vi "Periodic Tasks.vi"(8 "error in":errorcluster) -> ()   [LabVIEW 2012]
doc: "This VI runs in parallel to other tasks. It can contain as many user-defined periodic loops as you need. These can carry out PID or other sorts of timed response."
uses:
  <vilib>/Rock Robotics/SystemInterfaces/Utilities/FPGA_UtilitiesLED Source.ctl
  <vilib>/Rock Robotics/SystemInterfaces/Utilities/FPGA_UtilitiesLED State.ctl
  <vilib>/Rock Robotics/WPI/Relay/WPI_RelayValue.ctl
  <vilib>/Rock Robotics/WPI/RobotDrive/WPI_RobotDriveGetSetRefNum.vi
  Robot Global Data.vi
  <vilib>/Rock Robotics/WPI/Joystick/WPI_JoystickGetSetRefNum.vi
panel:
  out "end time":dbl
  out "start time":dbl
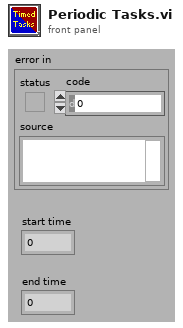
[diagram p1: front panel]
types:
  T1 = typedef "WPI_JoystickDevRef.ctl" = cluster{"Device":T2}
  T2 = typedef "WPI_JoystickDeviceEnum.ctl" = enum16{"USB 1", "USB 2", "USB 3", "USB 4", "Kinect 1", "Kinect 2"}
  T3 = typedef "WPI_RobotDriveDevRef.ctl" = cluster{"DevStatus":errorcluster, "Motors[]":T4[], "Square Inputs":bool, "Max Output":dbl, "Isochronous":bool}
  T4 = typedef "WPI_MotorControlDeviceRef.ctl" = cluster{"DeviceStatus":errorcluster, "Type":enum16{"PWM", "CAN"}, "PWM":cluster{"Digital Module":T5, "PWM Channel":T6, "DeadBand":T7}, "CAN":cluster{"Device Number":u8, "Control Mode":T8, "Semaphore":T9, "Max Vout":dbl}, "Invert":bool, "TransformRef":T10, "InvTransformRef":T10}
  T5 = typedef "FPGA_TypedefDigitalModule.ctl" = enum16{"Digital Module 1", "Digital Module 2"}
  T6 = typedef "FPGA_DIOPWMChannel.ctl" = enum8{"PWM 1", "PWM 2", "PWM 3", "PWM 4", "PWM 5", "PWM 6", "PWM 7", "PWM 8", "PWM 9", "PWM 10", "Invalid"}
  T7 = typedef "WPI_PWMDeadband.ctl" = cluster{"Name":string, "maxPositivePwm":i32, "minPositivePwm":i32, "centerPwm":i32, "maxNegativePwm":i32, "minNegativePwm":i32, "angularRange":u16}
  T8 = typedef "WPI_CANJaguar_ControlMode.ctl" = enum8{"Percent VBus", "Current", "Speed", "Position", "Voltage"}
  T9 = typedef "Semaphore RefNum" = refnum<k1>
  T10 = typedef "WPI_PWMTransform_ConPane.ctl" = refnum<vi>
  T11 = cluster{"JoystickDevRef":T1, "RobotDriveDevRef":T3}
  T12 = typedef "WPI_RelayValue.ctl" = enum16{"Off", "On", "Forward", "Reverse"}
  T13 = typedef "WPI_RelayDevRef.ctl" = cluster{"DevStatus":errorcluster, "Relay Channel":T14, "Digital Module":T5, "Relay Direction":T15}
  T14 = typedef "FPGA_DIORelayChannel.ctl" = enum8{"Relay 1", "Relay 2", "Relay 3", "Relay 4", "Relay 5", "Relay 6", "Relay 7", "Relay 8", "Invalid"}
  T15 = typedef "WPI_RelayDirection.ctl" = enum16{"Both directions", "Forward only", "Reverse only"}
  T16 = typedef "FPGA_UtilitiesLED State.ctl" = enum16{"Off", "On", "Toggle"}
  T17 = typedef "FPGA_UtilitiesLED Source.ctl" = enum16{"User LED", "FPGA LED"}
  T18 = typedef "WPI_CompressorDevRef.ctl" = cluster{"DevStatus":errorcluster, "DigitalInputDevRef":T19, "RelayDevRef":T13}
  T19 = typedef "WPI_DigitalInputDevRef.ctl" = cluster{"DevStatus":errorcluster, "DIO Channel":T20, "Digital Module":T5}
  T20 = typedef "FPGA_DIOChannel.ctl" = enum8{"DIO 1", "DIO 2", "DIO 3", "DIO 4", "DIO 5", "DIO 6", "DIO 7", "DIO 8", "DIO 9", "DIO 10", "DIO 11", "DIO 12", "DIO 13", "DIO 14", "Invalid"}
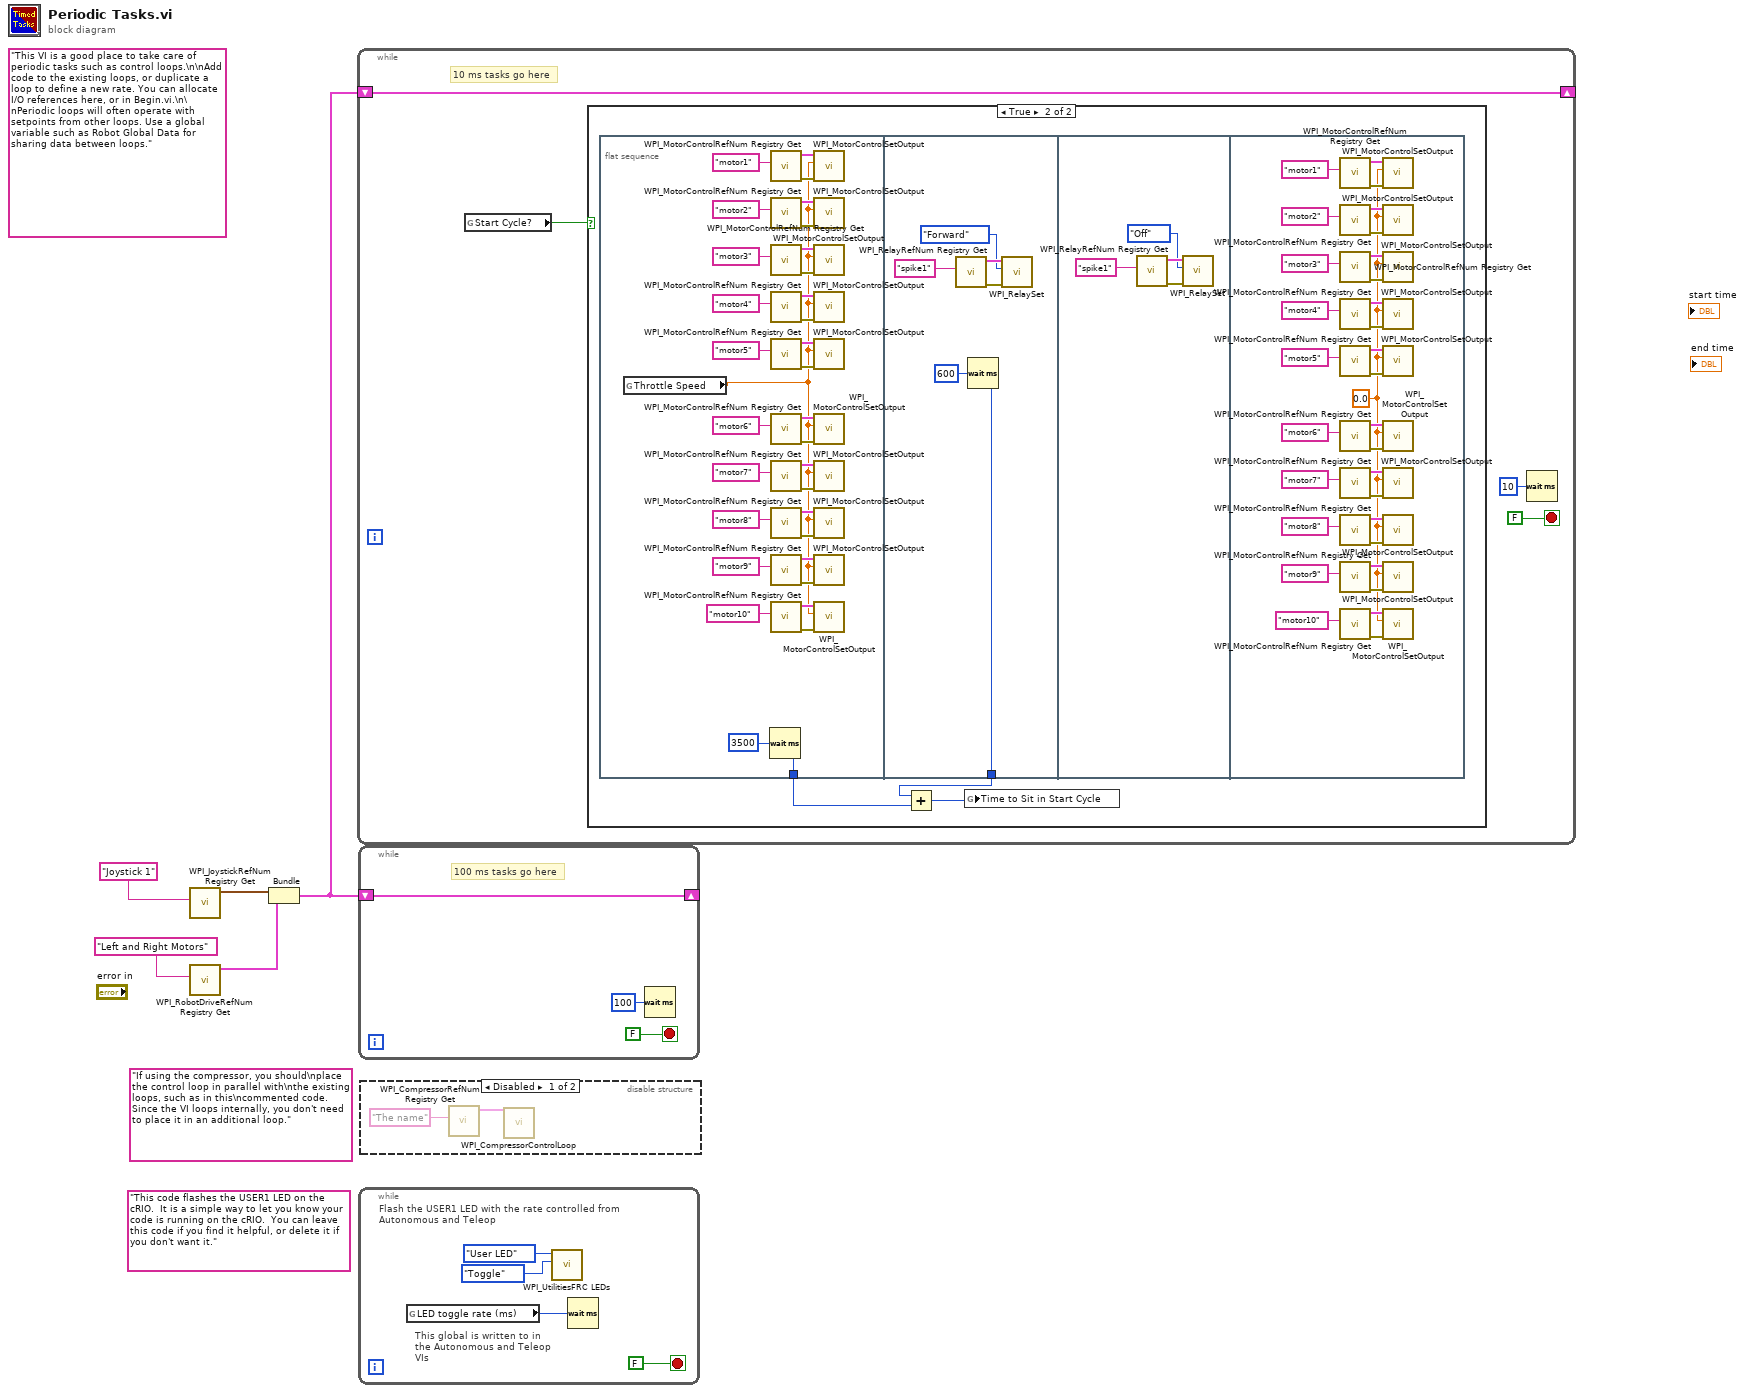
[diagram p0: block diagram]
diagram:
  (unwired) "If using the compressor, you should\nplace the control loop in parallel with\nthe existing loops, such as in this\ncommented code. Since the VI loops internally, you don't need to place it in an additional loop."
  (unwired) "This code flashes the USER1 LED on the cRIO.  It is a simple way to let you know your code is running on the cRIO.  You can leave this code if you find it helpful, or delete it if you don't want it."
  (unwired) "This VI is a good place to take care of periodic tasks such as control loops.\n\nAdd code to the existing loops, or duplicate a loop to define a new rate. You can allocate I/O references here, or in Begin.vi.\n\nPeriodic loops will often operate with setpoints from other loops. Use a global variable such as Robot Global Data for sharing data between loops."
  n1 = call <vilib>:"WPI_JoystickRefNum Registry Get.vi"("refnum name"="Joystick 1") -> ("JoystickDevRef"=w3:T1)  [unwired: 1 in, 9 out]
  n2 = call <vilib>:"WPI_RobotDriveRefNum Registry Get.vi"("refnum name"="Left and Right Motors") -> ("RobotDriveDevRef"=w2:T3)  [unwired: 1 in, 9 out]
  n3 = Bundle("JoystickDevRef"=w3, "RobotDriveDevRef"=w2) -> (w1:T11)  [unwired: 1 out]
  n4 = while {
    shift-right: [w7] -> _
    shift-left: w1 -> [w7]
    stop <- FALSE stop-if-true
    # "10 ms tasks go here"
    n5 = global read "Robot Global Data.vi" "Start Cycle?"() -> (w6:bool)
    n6 = case shown="True" w6 {
      frame False {
      }
      frame True {
        n7 = flat-sequence {
          tunnel: [w14] -> w10
          tunnel: [w46] -> w11
          frame #0 {
            n8 = global read "Robot Global Data.vi" "Throttle Speed"() -> (w13:dbl)
            n9 = Wait (ms)(milliseconds to wait=u32 3500) -> (millisecond timer value=w14:u32)
            n10 = call <vilib>:"WPI_MotorControlRefNum Registry Get.vi"("refnum name"="motor1") -> ("error out"=w40:errorcluster, "MotorControlDevRef"=w39:T4)  [unwired: 9 in]
            n11 = call <vilib>:"WPI_MotorControlRefNum Registry Get.vi"("refnum name"="motor2") -> ("error out"=w43:errorcluster, "MotorControlDevRef"=w42:T4)  [unwired: 9 in]
            n12 = call <vilib>:"WPI_MotorControlRefNum Registry Get.vi"("refnum name"="motor3") -> ("error out"=w34:errorcluster, "MotorControlDevRef"=w33:T4)  [unwired: 9 in]
            n13 = call <vilib>:"WPI_MotorControlRefNum Registry Get.vi"("refnum name"="motor4") -> ("error out"=w22:errorcluster, "MotorControlDevRef"=w21:T4)  [unwired: 9 in]
            n14 = call <vilib>:"WPI_MotorControlRefNum Registry Get.vi"("refnum name"="motor5") -> ("error out"=w25:errorcluster, "MotorControlDevRef"=w24:T4)  [unwired: 9 in]
            n15 = call <vilib>:"WPI_MotorControlRefNum Registry Get.vi"("refnum name"="motor6") -> ("error out"=w28:errorcluster, "MotorControlDevRef"=w27:T4)  [unwired: 9 in]
            n16 = call <vilib>:"WPI_MotorControlRefNum Registry Get.vi"("refnum name"="motor7") -> ("error out"=w16:errorcluster, "MotorControlDevRef"=w15:T4)  [unwired: 9 in]
            n17 = call <vilib>:"WPI_MotorControlRefNum Registry Get.vi"("refnum name"="motor8") -> ("error out"=w19:errorcluster, "MotorControlDevRef"=w18:T4)  [unwired: 9 in]
            n18 = call <vilib>:"WPI_MotorControlRefNum Registry Get.vi"("refnum name"="motor9") -> ("error out"=w37:errorcluster, "MotorControlDevRef"=w36:T4)  [unwired: 9 in]
            n19 = call <vilib>:"WPI_MotorControlRefNum Registry Get.vi"("refnum name"="motor10") -> ("error out"=w31:errorcluster, "MotorControlDevRef"=w30:T4)  [unwired: 9 in]
            n20 = call <vilib>:"WPI_MotorControlSetOutput.vi"("error in (no error)"=w40, "Output"=w13, "MotorControlDevRef"=w39) -> ()  [unwired: 6 in, 3 out]
            n21 = call <vilib>:"WPI_MotorControlSetOutput.vi"("error in (no error)"=w43, "Output"=w13, "MotorControlDevRef"=w42) -> ()  [unwired: 6 in, 3 out]
            n22 = call <vilib>:"WPI_MotorControlSetOutput.vi"("error in (no error)"=w34, "Output"=w13, "MotorControlDevRef"=w33) -> ()  [unwired: 6 in, 3 out]
            n23 = call <vilib>:"WPI_MotorControlSetOutput.vi"("error in (no error)"=w22, "Output"=w13, "MotorControlDevRef"=w21) -> ()  [unwired: 6 in, 3 out]
            n24 = call <vilib>:"WPI_MotorControlSetOutput.vi"("error in (no error)"=w25, "Output"=w13, "MotorControlDevRef"=w24) -> ()  [unwired: 6 in, 3 out]
            n25 = call <vilib>:"WPI_MotorControlSetOutput.vi"("error in (no error)"=w28, "Output"=w13, "MotorControlDevRef"=w27) -> ()  [unwired: 6 in, 3 out]
            n26 = call <vilib>:"WPI_MotorControlSetOutput.vi"("error in (no error)"=w16, "Output"=w13, "MotorControlDevRef"=w15) -> ()  [unwired: 6 in, 3 out]
            n27 = call <vilib>:"WPI_MotorControlSetOutput.vi"("error in (no error)"=w19, "Output"=w13, "MotorControlDevRef"=w18) -> ()  [unwired: 6 in, 3 out]
            n28 = call <vilib>:"WPI_MotorControlSetOutput.vi"("error in (no error)"=w37, "Output"=w13, "MotorControlDevRef"=w36) -> ()  [unwired: 6 in, 3 out]
            n29 = call <vilib>:"WPI_MotorControlSetOutput.vi"("error in (no error)"=w31, "Output"=w13, "MotorControlDevRef"=w30) -> ()  [unwired: 6 in, 3 out]
          }
          frame #1 {
            n30 = call <vilib>:"WPI_RelayRefNum Registry Get.vi"("refnum name"="spike1") -> ("error out"=w51:errorcluster, "RelayDevRef"=w50:T13)  [unwired: 9 in]
            n31 = Wait (ms)(milliseconds to wait=u32 600) -> (millisecond timer value=w46:u32)
            n32 = call <vilib>:"WPI_RelaySet.vi"("error in (no error)"=w51, "RelayValue"=WPI_RelayValue."Forward", "RelayDevRef"=w50) -> ()  [unwired: 7 in, 2 out]
          }
          frame #2 {
            n33 = call <vilib>:"WPI_RelayRefNum Registry Get.vi"("refnum name"="spike1") -> ("error out"=w55:errorcluster, "RelayDevRef"=w54:T13)  [unwired: 9 in]
            n34 = call <vilib>:"WPI_RelaySet.vi"("error in (no error)"=w55, "RelayValue"=WPI_RelayValue."Off", "RelayDevRef"=w54) -> ()  [unwired: 7 in, 2 out]
          }
          frame #3 {
            w56 = 0.0 ("f")
            n35 = call <vilib>:"WPI_MotorControlRefNum Registry Get.vi"("refnum name"="motor1") -> ("error out"=w82:errorcluster, "MotorControlDevRef"=w81:T4)  [unwired: 9 in]
            n36 = call <vilib>:"WPI_MotorControlRefNum Registry Get.vi"("refnum name"="motor2") -> ("error out"=w85:errorcluster, "MotorControlDevRef"=w84:T4)  [unwired: 9 in]
            n37 = call <vilib>:"WPI_MotorControlRefNum Registry Get.vi"("refnum name"="motor3") -> ("error out"=w76:errorcluster, "MotorControlDevRef"=w75:T4)  [unwired: 9 in]
            n38 = call <vilib>:"WPI_MotorControlRefNum Registry Get.vi"("refnum name"="motor4") -> ("error out"=w64:errorcluster, "MotorControlDevRef"=w63:T4)  [unwired: 9 in]
            n39 = call <vilib>:"WPI_MotorControlRefNum Registry Get.vi"("refnum name"="motor5") -> ("error out"=w67:errorcluster, "MotorControlDevRef"=w66:T4)  [unwired: 9 in]
            n40 = call <vilib>:"WPI_MotorControlRefNum Registry Get.vi"("refnum name"="motor6") -> ("error out"=w70:errorcluster, "MotorControlDevRef"=w69:T4)  [unwired: 9 in]
            n41 = call <vilib>:"WPI_MotorControlRefNum Registry Get.vi"("refnum name"="motor7") -> ("error out"=w58:errorcluster, "MotorControlDevRef"=w57:T4)  [unwired: 9 in]
            n42 = call <vilib>:"WPI_MotorControlRefNum Registry Get.vi"("refnum name"="motor8") -> ("error out"=w61:errorcluster, "MotorControlDevRef"=w60:T4)  [unwired: 9 in]
            n43 = call <vilib>:"WPI_MotorControlRefNum Registry Get.vi"("refnum name"="motor9") -> ("error out"=w79:errorcluster, "MotorControlDevRef"=w78:T4)  [unwired: 9 in]
            n44 = call <vilib>:"WPI_MotorControlRefNum Registry Get.vi"("refnum name"="motor10") -> ("error out"=w73:errorcluster, "MotorControlDevRef"=w72:T4)  [unwired: 9 in]
            n45 = call <vilib>:"WPI_MotorControlSetOutput.vi"("error in (no error)"=w82, "Output"=w56, "MotorControlDevRef"=w81) -> ()  [unwired: 6 in, 3 out]
            n46 = call <vilib>:"WPI_MotorControlSetOutput.vi"("error in (no error)"=w85, "Output"=w56, "MotorControlDevRef"=w84) -> ()  [unwired: 6 in, 3 out]
            n47 = call <vilib>:"WPI_MotorControlSetOutput.vi"("error in (no error)"=w76, "Output"=w56, "MotorControlDevRef"=w75) -> ()  [unwired: 6 in, 3 out]
            n48 = call <vilib>:"WPI_MotorControlSetOutput.vi"("error in (no error)"=w64, "Output"=w56, "MotorControlDevRef"=w63) -> ()  [unwired: 6 in, 3 out]
            n49 = call <vilib>:"WPI_MotorControlSetOutput.vi"("error in (no error)"=w67, "Output"=w56, "MotorControlDevRef"=w66) -> ()  [unwired: 6 in, 3 out]
            n50 = call <vilib>:"WPI_MotorControlSetOutput.vi"("error in (no error)"=w70, "Output"=w56, "MotorControlDevRef"=w69) -> ()  [unwired: 6 in, 3 out]
            n51 = call <vilib>:"WPI_MotorControlSetOutput.vi"("error in (no error)"=w58, "Output"=w56, "MotorControlDevRef"=w57) -> ()  [unwired: 6 in, 3 out]
            n52 = call <vilib>:"WPI_MotorControlSetOutput.vi"("error in (no error)"=w61, "Output"=w56, "MotorControlDevRef"=w60) -> ()  [unwired: 6 in, 3 out]
            n53 = call <vilib>:"WPI_MotorControlSetOutput.vi"("error in (no error)"=w79, "Output"=w56, "MotorControlDevRef"=w78) -> ()  [unwired: 6 in, 3 out]
            n54 = call <vilib>:"WPI_MotorControlSetOutput.vi"("error in (no error)"=w73, "Output"=w56, "MotorControlDevRef"=w72) -> ()  [unwired: 6 in, 3 out]
          }
        }
        n55 = Add(x=w11, y=w10) -> (x+y=w12:u32)
        n56 = global write "Robot Global Data.vi" "Time to Sit in Start Cycle"(w12) -> ()
      }
    }
    n57 = Wait (ms)(milliseconds to wait=u32 10) -> ()  [unwired: 1 out]
  }
  n58 = while {
    shift-right: [w87] -> _
    shift-left: w1 -> [w87]
    stop <- FALSE stop-if-true
    # "100 ms tasks go here"
    n59 = Wait (ms)(milliseconds to wait=u32 100) -> ()  [unwired: 1 out]
  }
  n60 = while {
    stop <- FALSE stop-if-true
    # "This global is written to in the Autonomous and Teleop VIs"
    # "Flash the USER1 LED with the rate controlled from Autonomous and Teleop"
    n61 = global read "Robot Global Data.vi" "LED toggle rate (ms)"() -> (w90:u32)
    n62 = call <vilib>:"WPI_UtilitiesFRC LEDs.vi"("State"=FPGA_UtilitiesLED_State."Toggle", "LED Type"=FPGA_UtilitiesLED_Source."User LED") -> ()  [unwired: 1 in, 9 out]
    n63 = Wait (ms)(milliseconds to wait=w90) -> ()  [unwired: 1 out]
  }
  n64 = disable-structure shown="Disabled" {
    frame Disabled {
      n65 = call <vilib>:"WPI_CompressorRefNum Registry Get.vi"("refnum name"="The name") -> ("CompressorDevRef"=w95:T18)  [unwired: 9 in, 1 out]
      n66 = call <vilib>:"WPI_CompressorControlLoop.vi"("CompressorDevRef"=w95) -> ()  [unwired: 11 in]
    }
    frame Enabled {
    }
  }
